vi "PuTTY.vi"() -> ()   [LabVIEW 2012]
panel:
  in  "Hide DOS\nWindow?":bool
  out "Command Executed":string
  out "Errors":string
  in  "Password":string="password"
  in  "Protocol":u16(ring)=2 items=["Telnet", "Rlogin", "SSH", "RAW"]
  in  "Host":string="host.domain.com"
  in  "Username":string="username"
  in  "Command(s) to Execute":string="pwd"
  out "Command Return Value(s)":string
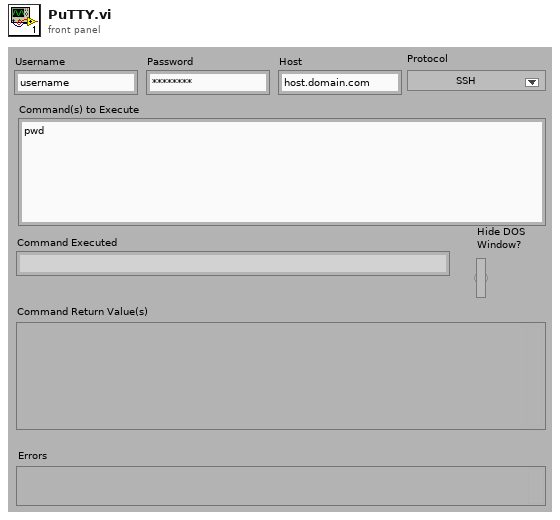
[diagram p1: front panel]
types:
  T1 = enum16{"open", "replace", "create", "open or create", "replace or create", "replace or create with confirmation"}
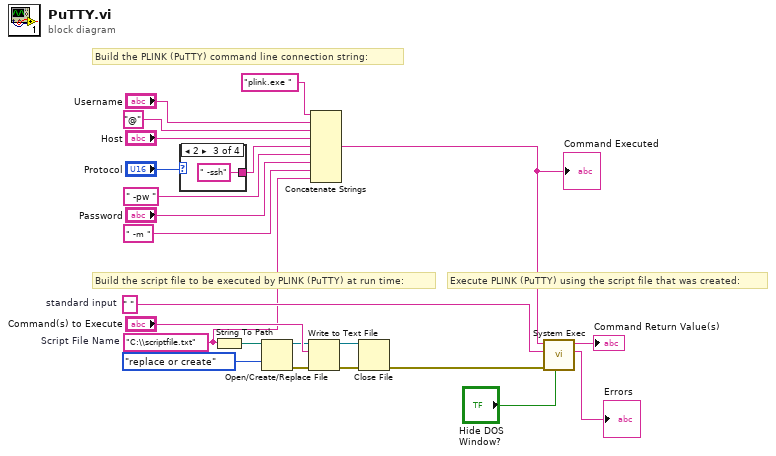
[diagram p0: block diagram]
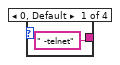
[diagram p2: hidden frame]
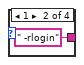
[diagram p3: hidden frame]
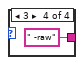
[diagram p4: hidden frame]
diagram:
  w15 = " "  # standard input
  w3 = "C:\\scriptfile.txt"  # Script File Name
  # "Execute PLINK (PuTTY) using the script file that was created:"
  # "Build the script file to be executed by PLINK (PuTTY) at run time:"
  # "Build the PLINK (PuTTY) command line connection string:"
  n1 = case shown="2" "Protocol" {
    tunnel: [" -telnet" " -rlogin" " -ssh" " -raw"] -> w9
    frame 0, Default {
    }
    frame 1 {
    }
    frame 2 {
    }
    frame 3 {
    }
  }
  n2 = String To Path(string=w3) -> (path=w4:path)
  n3 = Open/Create/Replace File(file path (use dialog)=w4, operation (0:open)=T1."replace or create") -> (refnum out=w18:refnum<file>, error out=w17:errorcluster)  [unwired: 4 in, 1 out]
  n4 = Write to Text File(file (use dialog)=w18, text="Command(s) to Execute", error in=w17) -> (refnum out=w21:refnum<file>, error out=w20:errorcluster)  [unwired: 2 out]
  n5 = Concatenate Strings("plink.exe " ("command line"), "Username", "@" ("string"), "Host", w9, " -pw " ("string"), "Password", " -m " ("string"), w3) -> (w5:string)
  "Command Executed" <- w5
  n6 = Close File(refnum=w21, error in=w20) -> (error out=w19:errorcluster)  [unwired: 1 out]
  n7 = call <vilib>:"System Exec.vi"("run minimized? (F)"="Hide DOS\nWindow?", "error in (no error)"=w19, "standard input"=w15, "command line"=w5) -> ("standard error"=→"Errors":string, "standard output"=→"Command Return Value(s)":string)  [unwired: 2 in, 4 out]
